vi "EnvFloRead.vi"(8 "error in (no error)":errorcluster, 10 "read byte count":u32, 11 "VISA Refnum in":refnum<visa-resource-name>) -> (0 "error out":errorcluster, 1 "value":dbl, 2 "read buffer":string, 3 "VISA Refnum out":refnum<visa-resource-name>, 4 "timestamp":string, 5 "return count":u32)   [LabVIEW 2016]
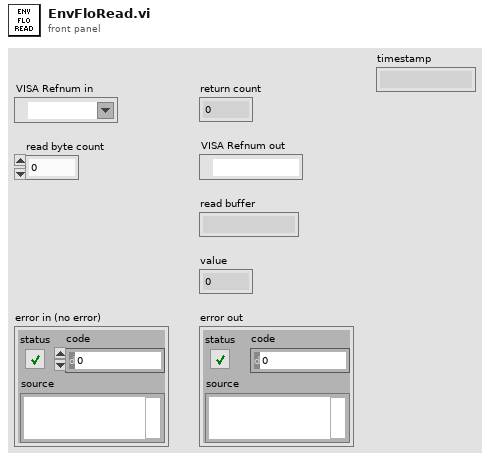
[diagram p1: front panel]
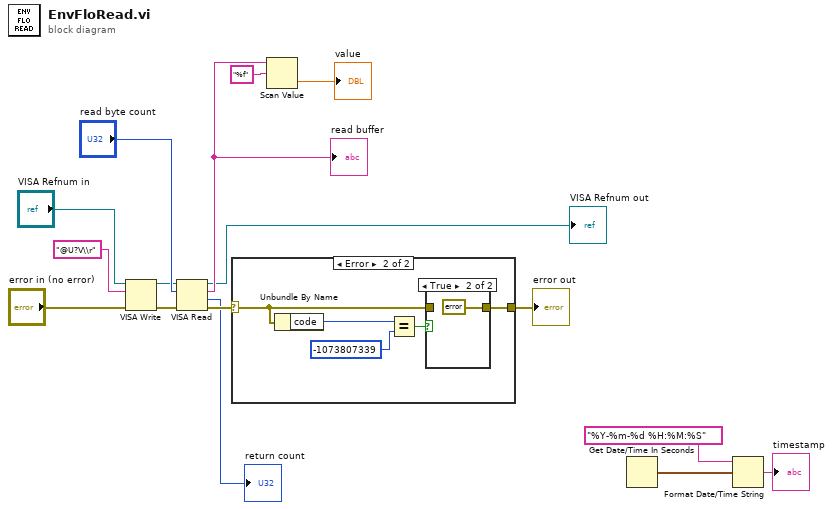
[diagram p0: block diagram]
diagram:
  n1 = VISA Write(VISA resource name="VISA Refnum in", write buffer="@U?V\\r", error in (no error)="error in (no error)") -> (VISA resource name out=w7:refnum<visa-resource-name>, error out=w8:errorcluster)  [unwired: 1 out]
  n2 = VISA Read(VISA resource name=w7, byte count="read byte count", error in (no error)=w8) -> (VISA resource name out=→"VISA Refnum out":refnum<visa-resource-name>, read buffer=w14:string, return count=→"return count":u32, error out=w12:errorcluster)
  "read buffer" <- w14
  n3 = case shown="Error" w12 {
    selector: w12 -> [w17 w18]
    tunnel: [w17 w19] -> w13
    frame No Error {
    }
    frame Error {
      n4 = Unbundle By Name(w18) -> ("code"=w22:i32)
      n5 = Equal?(x=w22, y=-1073807339) -> (x = y?=w20:bool)
      n6 = case shown="True" w20 {
        tunnel: [w23 errorcluster {"status"=FALSE, "code"=0, "source"=""} ("error constant")] -> w19
        tunnel: w18 -> [w23 _]
        frame False {
        }
        frame True {
        }
      }
    }
  }
  "error out" <- w13
  n7 = Scan Value(string=w14, format string="%f") -> (value=→"value":dbl)  [unwired: 1 in, 1 out]
  n8 = Get Date/Time In Seconds() -> (seconds since 1Jan1904=w3:timestamp)
  n9 = Format Date/Time String(time format string (%c)="%Y-%m-%d %H:%M:%S", seconds (now)=w3) -> (date/time string=→"timestamp":string)  [unwired: 1 in]
